vi "CMD_DBLOGOUT.vi"(6 "Gantry in":refnum<class "Gantry.lvclass">, 8 "error in (no error)":errorcluster, 10 "Arguments":string[](array[string]), 11 "gScript Interpreter in":refnum<class "gScript Interpreter.lvclass">) -> (0 "error out":errorcluster, 3 "gScript Interpreter out":refnum<class "gScript Interpreter.lvclass">, 4 "Gantry out":refnum<class "Gantry.lvclass">)   [LabVIEW 2017, in "gScript Interpreter.lvclass"]
uses:
  gScript Interpreter.lvclass
  Shared Components/Gantry Class/Gantry.lvclass
  Shared Components/FlexWorktable/FlexWorktable.lvclass
  Shared Components/External/Database/Database.lvlib
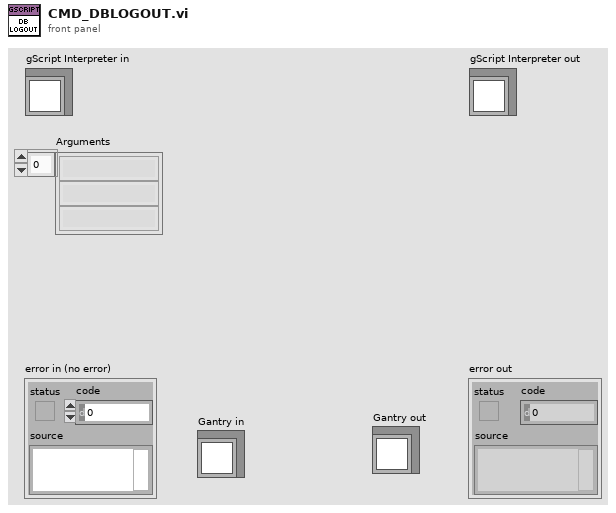
[diagram p1: front panel]
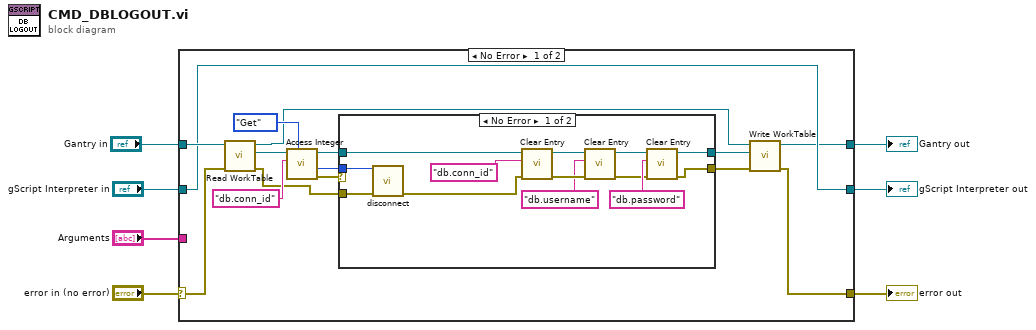
[diagram p0: block diagram]
diagram:
  n1 = case shown="No Error" "error in (no error)" {
    selector: "error in (no error)" -> [w21 w40]
    tunnel: [w8 w40] -> w6
    tunnel: [w10 w39] -> w4
    tunnel: "gScript Interpreter in" -> [w10 w39]
    tunnel: "Arguments" -> [_ _]
    tunnel: "Gantry in" -> [w22 w38]
    tunnel: [w9 w38] -> w1
    frame No Error {
      n2 = call-dynamic "Read WorkTable.vi"("error in"=w21, "Gantry Class in"=w22) -> ("error out"=w11:errorcluster, "Worktable"=w20:refnum<class "FlexWorktable.lvclass">, "Gantry Class out"=w14:refnum<class "Gantry.lvclass">)  [unwired: 7 in]
      n3 = call-dynamic "Access Integer.vi"("Get/Set"=enum16{"Get", "Set"}."Get", "Key"="db.conn_id", "FlexWorktable in"=w20) -> ("error out"=w17:errorcluster, "Value out"=w15:i32, "FlexWorktable out"=w16:refnum<class "FlexWorktable.lvclass">)  [unwired: 6 in]
      n4 = case shown="No Error" w17 {
        tunnel: w16 -> [w34 w37]
        tunnel: w15 -> [w35 _]
        tunnel: [w25 w37] -> w13
        tunnel: [w24 w36] -> w12
        tunnel: w11 -> [w23 w36]
        frame No Error {
          n5 = call "disconnect.vi"("DB Session ID"=w35, "error in (no error)"=w23) -> ("error out"=w33:errorcluster)  [unwired: 13 in]
          n6 = call "Clear Entry.vi"("error in (no error)"=w33, "Key"="db.conn_id", "FlexWorktable in"=w34) -> ("error out"=w30:errorcluster, "FlexWorktable out"=w31:refnum<class "FlexWorktable.lvclass">)  [unwired: 6 in, 1 out]
          n7 = call "Clear Entry.vi"("error in (no error)"=w30, "Key"="db.username", "FlexWorktable in"=w31) -> ("error out"=w26:errorcluster, "FlexWorktable out"=w28:refnum<class "FlexWorktable.lvclass">)  [unwired: 6 in, 1 out]
          n8 = call "Clear Entry.vi"("error in (no error)"=w26, "Key"="db.password", "FlexWorktable in"=w28) -> ("error out"=w24:errorcluster, "FlexWorktable out"=w25:refnum<class "FlexWorktable.lvclass">)  [unwired: 6 in, 1 out]
        }
        frame Error {
        }
      }
      n9 = call-dynamic "Write WorkTable.vi"("error in (no error)"=w12, "FlexWorktable"=w13, "Gantry Class in"=w14) -> ("error out"=w8:errorcluster, "Gantry Class out"=w9:refnum<class "Gantry.lvclass">)  [unwired: 7 in]
    }
    frame Error {
    }
  }
  "error out" <- w6
  "gScript Interpreter out" <- w4
  "Gantry out" <- w1
